vi "Fetch (Measurements).vi"(0 "VISA resource name":refnum<visa-resource-name>, 5 "Timeout (10000 ms)":i32=10000 format="%#.6g", 7 "Buffer Name (defbuffer1)":string="defbuffer1", 9 "Buffer Elements":string="READ", 11 "error in (no error)":errorcluster) -> (4 "VISA resource name out":refnum<visa-resource-name>, 6 "Data out":string, 15 "error out":errorcluster)   [LabVIEW 2018, in "Keithley 2450.lvlib"]
doc: "Fetches data for voltage, current, resistance, timestamp, and status. These readings are then provided in separate arrays for each type of reading.\n\nBuffer Element can be a single parameter or multiple parameters.Parameters have to be separated by comma followed by space.(eg - READ, SEC, DATE)\n\n<B>Note</B> Use this VI only with other low-level VIs. The high-level VIs automatically incorporate this functionality. This VI does not check the instrument status. If you want to check the instrument status, call the Error Query VI at the conclusion of the sequence."
uses:
  <instrlib>/Keithley 2450/Keithley 2450.lvlib
panel:
  out "Status":sgl[](array[numeric])
  out "Timestamp":sgl[](array[numeric])
  out "Resistance":sgl[](array[numeric])
  out "Current":sgl[](array[numeric])
  out "Voltage":sgl[](array[numeric])
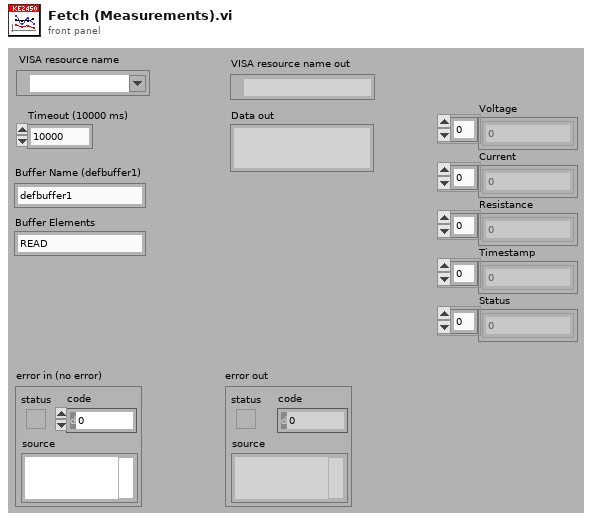
[diagram p1: front panel]
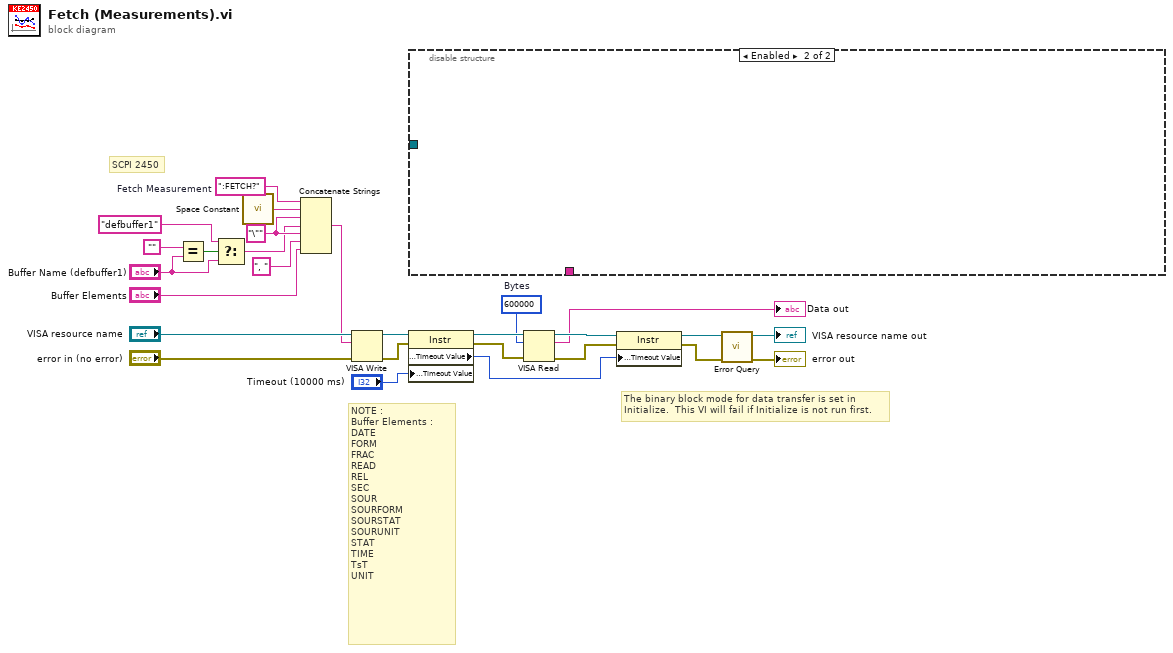
[diagram p0: block diagram]
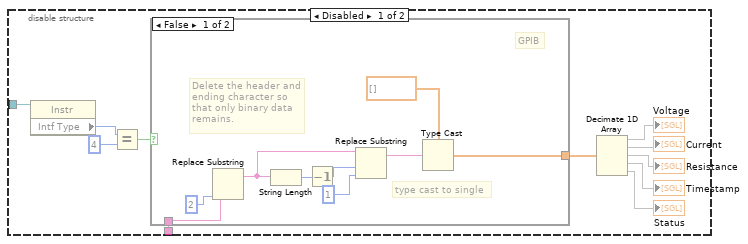
[diagram p2: hidden frame]
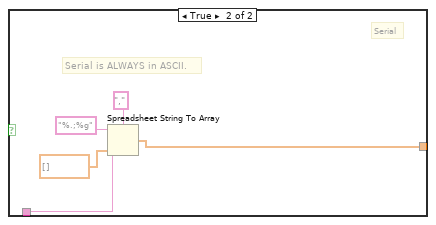
[diagram p3: hidden frame]
diagram:
  w10 = "\""
  w7 = ":FETCH?"  # Fetch Measurement
  w17 = u32 600000  # Bytes
  # "NOTE :\nBuffer Elements :\nDATE\nFORM\nFRAC\nREAD\nREL\nSEC\nSOUR\nSOURFORM\nSOURSTAT\nSOURUNIT\nSTAT\nTIME\nTsT\nUNIT"
  # "SCPI 2450"
  # "The binary block mode for data transfer is set in Initialize.  This VI will fail if Initialize is not run first."
  n1 = Equal?(x="", y="Buffer Name (defbuffer1)") -> (x = y?=w13:bool)
  n2 = Select(t="defbuffer1", s=w13, f="Buffer Name (defbuffer1)") -> (s? t:f=w9:string)
  n3 = call <vilib>:"Space Constant.vi"() -> ("String"=w8:string)
  n4 = Concatenate Strings(w7, w8, w10, w9, w10, ", " ("string"), "Buffer Elements") -> (w25:string)
  n5 = VISA Write(VISA resource name="VISA resource name", write buffer=w25, error in (no error)="error in (no error)") -> (VISA resource name out=w15:refnum<visa-resource-name>, error out=w24:errorcluster)  [unwired: 1 out]
  n6 = property class="Instr"(reference=w15, error in=w24, "General Settings:Timeout Value"="Timeout (10000 ms)") -> (reference out=w23:refnum<visa-resource-name>, error out=w22:errorcluster, "General Settings:Timeout Value"=w18:u32)
  n7 = disable-structure shown="Enabled" {
    disable-tunnel: _ -> [w38 _]
    disable-tunnel: _ -> [w31 _]
    frame Disabled {
      n8 = property class="Instr"(reference=w31) -> ("Intf Type"=w30:u16)  [unwired: 1 in, 2 out]
      n9 = Equal?(x=w30, y=u16 4) -> (x = y?=w28:bool)
      n10 = case shown="False" w28 {
        tunnel: w38 -> [w47 w52]
        tunnel: [w39 w48] -> w37
        frame False {
          # "Delete the header and ending character so that only binary data remains."
          # "GPIB"
          # "type cast to single"
          n11 = Replace Substring(2:2 ("length (len. of substring)"), 5:w47) -> (1:w45:string)  [unwired: 3 out]
          n12 = String Length(string=w45) -> (length=w44:i32)
          n13 = Decrement(x=w44) -> (x-1=w43:i32)
          n14 = Replace Substring(2:1 ("length (len. of substring)"), 3:w43, 5:w45) -> (1:w41:string)  [unwired: 2 out]
          n15 = Type Cast(type=sgl[] [], x=w41) -> (*(type *) &x=w39:sgl[])
        }
        frame True {
          # "Serial is ALWAYS in ASCII."
          # "Serial"
          n16 = Spreadsheet String To Array(delimiter (Tab)=",", format string="%.;%g", spreadsheet string=w52, array type (2D Dbl)=sgl[] []) -> (array=w48:sgl[])
        }
      }
      n17 = Decimate 1D Array(w37) -> (→"Voltage":sgl[], →"Current":sgl[], →"Resistance":sgl[], →"Timestamp":sgl[], →"Status":sgl[])
    }
    frame Enabled {
    }
  }
  n18 = VISA Read(VISA resource name=w23, byte count=w17, error in (no error)=w22) -> (VISA resource name out=w20:refnum<visa-resource-name>, read buffer=→"Data out":string, error out=w19:errorcluster)  [unwired: 1 out]
  n19 = property class="Instr"(reference=w20, error in=w19, "General Settings:Timeout Value"=w18) -> (reference out=w6:refnum<visa-resource-name>, error out=w4:errorcluster)
  n20 = call <instrlib>:"Error Query.vi"("error in (no error)"=w4, "VISA resource name"=w6) -> ("error out"=→"error out":errorcluster, "VISA resource name out"=→"VISA resource name out":refnum<visa-resource-name>)  [unwired: 8 out]
